vi "Lift.vi"() -> ()   [LabVIEW 2018]
uses:
  <vilib>/Rock Robotics/WPI/ThirdParty/Phoenix-LabVIEW/Motor Controller/Controls/CTRE_Phoenix_MotorControl_ControlMode.ctl
  Lift Global.vi
  Times/Times Global.vi
  <vilib>/addons/control/pid/pid.llb/PID (DBL).vi
  <vilib>/Rock Robotics/WPI/ThirdParty/Phoenix-LabVIEW/Motor Controller/Get/CTRE_Phoenix_MotorController_GetSelectedSensorData.vi
  Cargo Intake/Cargo Intake Global.vi
  <vilib>/addons/control/pid/NI_PID_pid.lvlib
  <vilib>/Rock Robotics/WPI/Counter/WPI_CounterDigitalInputToDigitalSource.vi
  <vilib>/Rock Robotics/SystemInterfaces/DIO/FPGA_DIOChannel.ctl
panel:
  in  "Zero":bool
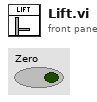
[diagram p1: front panel]
types:
  T1 = typedef "FPGA_DIOChannel.ctl" = enum8{"DIO 0", "DIO 1", "DIO 2", "DIO 3", "DIO 4", "DIO 5", "DIO 6", "DIO 7", "DIO 8", "DIO 9", "DIO MXP 0", "DIO MXP 1", "DIO MXP 2", "DIO MXP 3", "DIO MXP 4", "DIO MXP 5", "DIO MXP 6", "DIO MXP 7", "DIO MXP 8", "DIO MXP 9", "DIO MXP 10", "DIO MXP 11", "DIO MXP 12", "DIO MXP 13", "DIO MXP 14", "DIO MXP 15", "SPI Port CS1", "SPI Port CS2", "SPI Port CS3", "SPI Port MISO", "SPI Port MOSI", "Invalid"}
  T2 = typedef "WPI_DigitalInputDevRef.ctl" = cluster{"DevStatus":errorcluster, "DIO Channel":T1}
  T3 = typedef "FPGA_CounterEncoderSourceConvertionLVSourceType.ctl" = cluster{"DevStatus":errorcluster, "AnalogTriggerMode?":bool, "DigitalMode":cluster{"DIO Channel":T4}, "AnalogTriggerMode":cluster{"AnalogTriggerIndex":T5, "OutputType":T6}}
  T4 = typedef "FPGA_DIODigitalSourceChannel.ctl" = enum8{"DIO 0", "DIO 1", "DIO 2", "DIO 3", "DIO 4", "DIO 5", "DIO 6", "DIO 7", "DIO 8", "DIO 9", "DIO MXP 0", "DIO MXP 1", "DIO MXP 2", "DIO MXP 3", "DIO MXP 4", "DIO MXP 5", "DIO MXP 6", "DIO MXP 7", "DIO MXP 8", "DIO MXP 9", "DIO MXP 10", "DIO MXP 11", "DIO MXP 12", "DIO MXP 13", "DIO MXP 14", "DIO MXP 15", "SPI Port CS1", "SPI Port CS2", "SPI Port CS3", "SPI Port MISO", "SPI Port MOSI", "Disabled"}
  T5 = typedef "FPGA_AnalogTriggerIndex.ctl" = enum8{"Trig 0", "Trig 1", "Trig 2", "Trig 3", "Trig 4", "Trig 5", "Trig 6", "Trig 7", "Invalid"}
  T6 = typedef "FPGA_AnalogTriggerOutType.ctl" = enum16{"InWindow", "TriggerState", "Rising", "Falling"}
  T7 = typedef "WPI_EncoderDevRef.ctl" = cluster{"DevStatus":errorcluster, "EncoderIndex":T8, "CounterIndex":T9, "DistancePerCount":dbl, "Decoding Type":T10}
  T8 = typedef "FPGA_EncoderIdx.ctl" = enum8{"Enc 0", "Enc 1", "Enc 2", "Enc 3", "Enc 4", "Enc 5", "Enc 6", "Enc 7", "Invalid"}
  T9 = typedef "FPGA_CounterCtrSystemIndex.ctl" = enum8{"Ctr 0", "Ctr 1", "Ctr 2", "Ctr 3", "Ctr 4", "Ctr 5", "Ctr 6", "Ctr 7", "Invalid"}
  T10 = typedef "WPI_EncoderType.ctl" = enum16{"1x", "2x", "4x"}
  T11 = enum16{"Ultra Manual Control", "Manual Control", "Basic Control", "Automated Control", "Autonomous Control"}
  T12 = enum16{"N/A", "Hatch Panel Zone 1", "Hatch Panel Zone 2", "Hatch Panel Zone 3", "Cargo Zone 1", "Cargo Zone 2", "Cargo Zone 3"}
  T13 = typedef "WPI_MotorControlDeviceRef.ctl" = cluster{"DeviceStatus":errorcluster, "Type":T14, "PWM":cluster{"PWM Channel":T15, "DeadBand":T16}, "CAN":cluster{"Device Number":u8, "SetOutput VI Ref":variant, "GetOutput VI Ref":variant, "Enable VI Ref":variant, "Disable VI Ref":variant, "Data":variant}, "Invert":bool, "DIO PWM":cluster{"PWM \"Enable\" Channel":T15, "DIOChannel":T1, "PWM Rate":dbl}}
  T14 = typedef "WPI_MotorControlType.ctl" = enum16{"PWM", "CAN", "DIO PWM"}
  T15 = typedef "FPGA_DIOPWMChannel.ctl" = enum8{"PWM 0", "PWM 1", "PWM 2", "PWM 3", "PWM 4", "PWM 5", "PWM 6", "PWM 7", "PWM 8", "PWM 9", "PWM MXP 0", "PWM MXP 1", "PWM MXP 2", "PWM MXP 3", "PWM MXP 4", "PWM MXP 5", "PWM MXP 6", "PWM MXP 7", "PWM MXP 8", "PWM MXP 9", "Invalid"}
  T16 = typedef "WPI_PWMDeadband.ctl" = cluster{"Name":string, "maxPositivePwm":i32, "minPositivePwm":i32, "centerPwm":i32, "maxNegativePwm":i32, "minNegativePwm":i32, "angularRange":u16}
  T17 = typedef "CTRE_Phoenix_MotorControl_ControlMode.ctl" = u16
  T18 = typedef "Control 3.ctl" = dbl
  T19 = cluster{"proportional gain (Kc)":dbl, "integral time(Ti, min)":dbl, "derivative time(Td, min) 2":dbl}
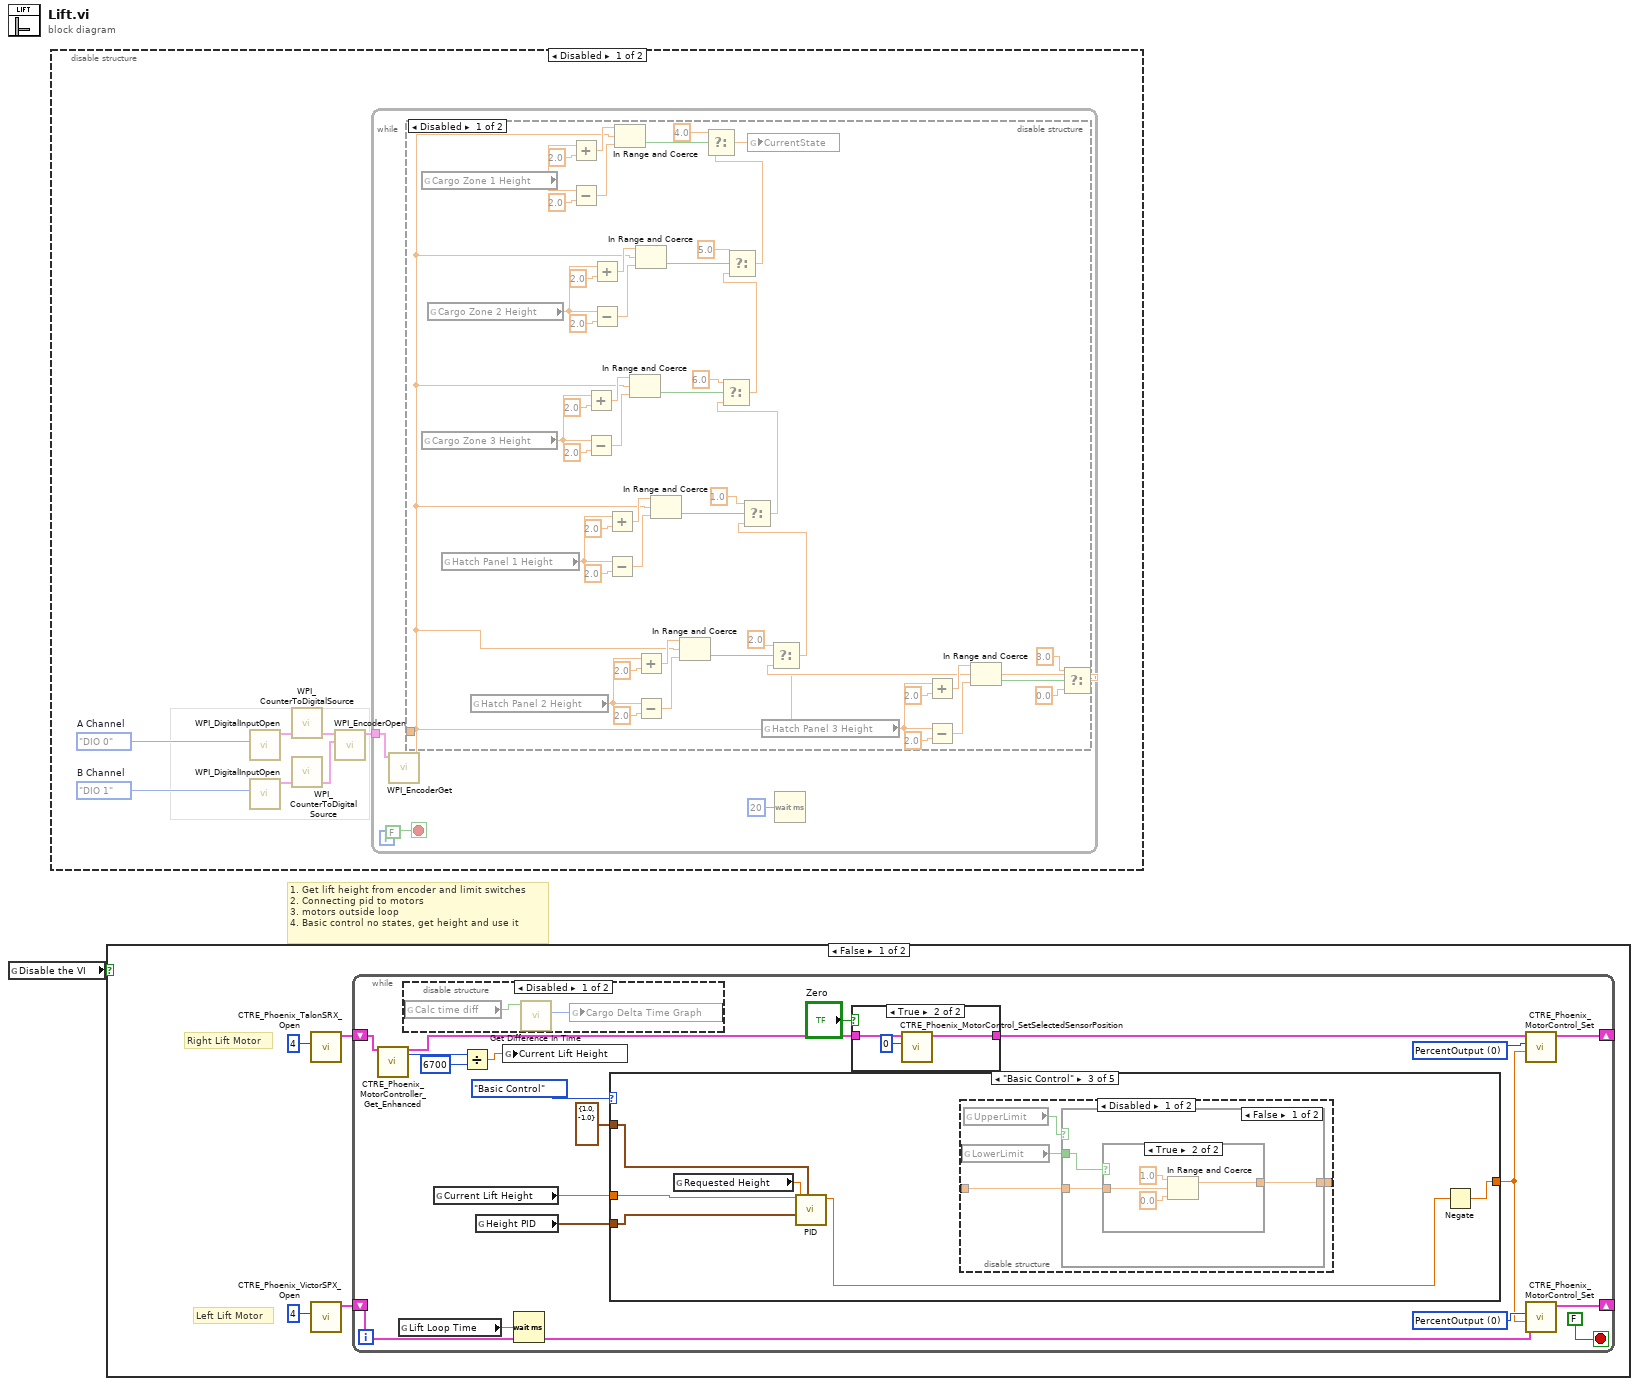
[diagram p0: block diagram]
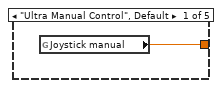
[diagram p6: hidden frame]
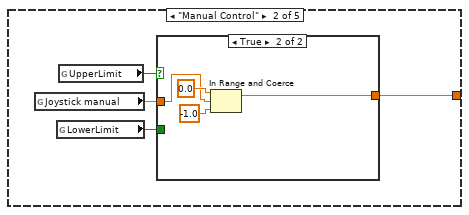
[diagram p7: hidden frame]
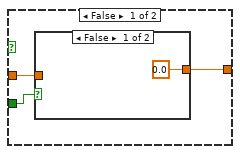
[diagram p8: hidden frame]
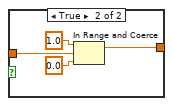
[diagram p9: hidden frame]
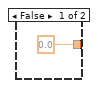
[diagram p10: hidden frame]
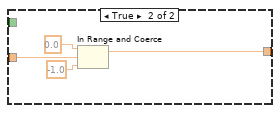
[diagram p11: hidden frame]
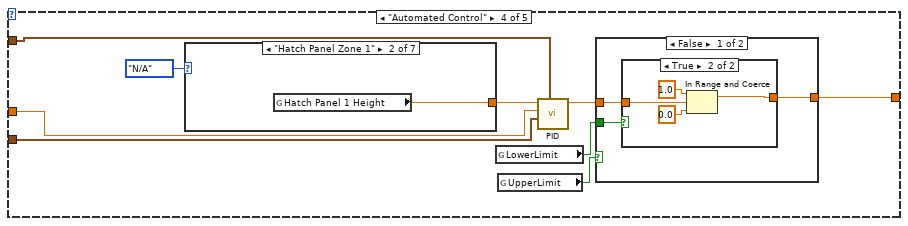
[diagram p13: hidden frame]
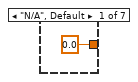
[diagram p14: hidden frame]
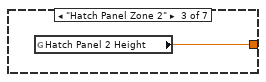
[diagram p15: hidden frame]
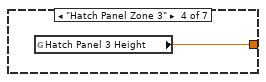
[diagram p16: hidden frame]
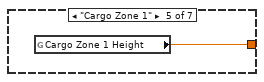
[diagram p17: hidden frame]
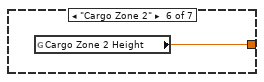
[diagram p18: hidden frame]
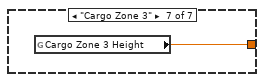
[diagram p19: hidden frame]
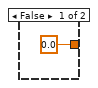
[diagram p20: hidden frame]
diagram:
  # "1. Get lift height from encoder and limit switches\n2. Connecting pid to motors\n3. motors outside loop\n4. Basic control no states, get height and use it"
  n1 = global read "Lift Global.vi" "Disable the VI"() -> (w1:bool)
  n2 = disable-structure shown="Disabled" {
    frame Disabled {
      w8 = FPGA_DIOChannel."DIO 1"  # B Channel
      w7 = FPGA_DIOChannel."DIO 0"  # A Channel
      n3 = call <vilib>:"WPI_DigitalInputOpen.vi"("DIO Channel"=w7) -> ("DigitalInputDevRef"=w4:T2)  [unwired: 1 in, 9 out]
      n4 = call <vilib>:"WPI_DigitalInputOpen.vi"("DIO Channel"=w8) -> ("DigitalInputDevRef"=w5:T2)  [unwired: 1 in, 9 out]
      n5 = call-poly <vilib>:"WPI_CounterToDigitalSource.vi"("DigitalInputDevRef"=w4) -> ("Digital Source"=w3:T3)  [unwired: 6 out]
      n6 = call-poly <vilib>:"WPI_CounterToDigitalSource.vi"("DigitalInputDevRef"=w5) -> ("Digital Source"=w6:T3)  [unwired: 6 out]
      n7 = call <vilib>:"WPI_EncoderOpen.vi"("BSource"=w6, "ASource"=w3) -> ("EncoderDevRef"=w2:T7)  [unwired: 6 in, 3 out]
      n8 = while {
        tunnel: w2 -> [w12]
        stop <- FALSE stop-if-true
        n9 = call <vilib>:"WPI_EncoderGet.vi"("EncoderDevRef"=w12) -> ("Distance"=w10:dbl)  [unwired: 5 in, 5 out]
        n10 = disable-structure shown="Disabled" {
          disable-tunnel: w10 -> [w13 _]
          frame Disabled {
            n11 = global read "Lift Global.vi" "Cargo Zone 1 Height"() -> (w53:dbl)
            n12 = global read "Lift Global.vi" "Cargo Zone 3 Height"() -> (w41:dbl)
            n13 = global read "Lift Global.vi" "Cargo Zone 2 Height"() -> (w59:dbl)
            n14 = global read "Lift Global.vi" "Hatch Panel 1 Height"() -> (w47:dbl)
            n15 = global read "Lift Global.vi" "Hatch Panel 2 Height"() -> (w29:dbl)
            n16 = Add(x=w53, y=2.0) -> (x+y=w55:dbl)
            n17 = Subtract(x=w53, y=2.0) -> (x-y=w56:dbl)
            n18 = Add(x=w41, y=2.0) -> (x+y=w43:dbl)
            n19 = Subtract(x=w41, y=2.0) -> (x-y=w44:dbl)
            n20 = Add(x=w59, y=2.0) -> (x+y=w61:dbl)
            n21 = Subtract(x=w59, y=2.0) -> (x-y=w62:dbl)
            n22 = Add(x=w47, y=2.0) -> (x+y=w49:dbl)
            n23 = Subtract(x=w47, y=2.0) -> (x-y=w50:dbl)
            n24 = In Range and Coerce(upper limit=w55, x=w13, lower limit=w56) -> (In Range?=w51:bool)  [unwired: 1 out]
            n25 = In Range and Coerce(upper limit=w43, x=w13, lower limit=w44) -> (In Range?=w39:bool)  [unwired: 1 out]
            n26 = In Range and Coerce(upper limit=w61, x=w13, lower limit=w62) -> (In Range?=w57:bool)  [unwired: 1 out]
            n27 = Add(x=w29, y=2.0) -> (x+y=w31:dbl)
            n28 = Subtract(x=w29, y=2.0) -> (x-y=w32:dbl)
            n29 = In Range and Coerce(upper limit=w49, x=w13, lower limit=w50) -> (In Range?=w45:bool)  [unwired: 1 out]
            n30 = In Range and Coerce(upper limit=w31, x=w13, lower limit=w32) -> (In Range?=w27:bool)  [unwired: 1 out]
            n31 = global read "Lift Global.vi" "Hatch Panel 3 Height"() -> (w35:dbl)
            n32 = Add(x=w35, y=2.0) -> (x+y=w37:dbl)
            n33 = Subtract(x=w35, y=2.0) -> (x-y=w38:dbl)
            n34 = In Range and Coerce(upper limit=w37, x=w13, lower limit=w38) -> (In Range?=w33:bool)  [unwired: 1 out]
            n35 = Select(t=3.0, s=w33, f=0.0 ("t")) -> (s? t:f=w23:dbl)
            n36 = Select(t=2.0, s=w27, f=w23) -> (s? t:f=w24:dbl)
            n37 = Select(t=1.0, s=w45, f=w24) -> (s? t:f=w25:dbl)
            n38 = Select(t=6.0, s=w39, f=w25) -> (s? t:f=w26:dbl)
            n39 = Select(t=5.0, s=w57, f=w26) -> (s? t:f=w20:dbl)
            n40 = Select(t=4.0, s=w51, f=w20) -> (s? t:f=w21:dbl)
            n41 = global write "Lift Global.vi" "CurrentState"(w21) -> ()
          }
          frame Enabled {
          }
        }
        n42 = Wait (ms)(milliseconds to wait=u32 20) -> ()  [unwired: 1 out]
      }
    }
    frame Enabled {
    }
  }
  n43 = case shown="False" w1 {
    frame False {
      # "Left Lift Motor"
      # "Right Lift Motor"
      n44 = call <vilib>:"CTRE_Phoenix_TalonSRX_Open.vi"("Device Number"=u8 4) -> ("CAN Talon SRX Ref"=w66:T13)  [unwired: 9 in, 1 out]
      n45 = call <vilib>:"CTRE_Phoenix_VictorSPX_Open.vi"("Device Number"=u8 4) -> ("CAN Talon SRX Ref"=w64:T13)  [unwired: 9 in, 1 out]
      n46 = while {
        shift-right: [w81] -> _
        shift-left: w66 -> [w73]
        shift-right: [w79] -> _
        shift-left: w64 -> [w78]
        stop <- FALSE stop-if-true
        w80 = T17 0 items=["PercentOutput"=0, "Position"=1, "Velocity"=2, "Current"=3, "Follower"=5, "MotionProfile"=6, "MotionMagic"=7, "MotionProfileArc"=10, "Disabled"=15] ("Control Mode")
        w82 = T17 0 items=["PercentOutput"=0, "Position"=1, "Velocity"=2, "Current"=3, "Follower"=5, "MotionProfile"=6, "MotionMagic"=7, "MotionProfileArc"=10, "Disabled"=15] ("Control Mode")
        n47 = call-poly <vilib>:"CTRE_Phoenix_MotorController_Get_Enhanced.vi"("PhoenixMotorControlDevRef"=w73) -> ("PhoenixMotorControlDevRef"=w72:T13, "Position (Raw Sensor Units)"=w69:i32)  [unwired: 11 in, 2 out]
        n48 = global read "Times Global.vi" "Lift Loop Time"() -> (w85:T18)
        n49 = disable-structure shown="Disabled" {
          frame Disabled {
            n50 = global read "Cargo Intake Global.vi" "Calc time diff"() -> (w91:bool)
            n51 = call "Get Difference In Time.vi"("Calculate Time Difference"=w91) -> ("Delta Time over Time"=w90:u32)  [unwired: 9 in, 1 out]
            n52 = global write "Times Global.vi" "Cargo Delta Time Graph"(w90) -> ()
          }
          frame Enabled {
          }
        }
        n53 = global read "Lift Global.vi" "Current Lift Height"() -> (w74:dbl)
        n54 = Divide(x=w69, y=6700) -> (x/y=w68:dbl)
        n55 = global read "Lift Global.vi" "Height PID"() -> (w75:T19)
        n56 = global write "Lift Global.vi" "Current Lift Height"(w68) -> ()
        n57 = Wait (ms)(milliseconds to wait=w85) -> ()  [unwired: 1 out]
        n58 = case shown="\"Basic Control\"" T11."Basic Control" ("LiftMode") {
          tunnel: [w92 w93 w110 w136 0.0 ("Cargo Zone 3 Height")] -> w77
          tunnel: w74 -> [_ _ w114 w134 _]
          tunnel: w75 -> [_ _ w113 w133 _]
          tunnel: cluster{"output high":dbl, "output low":dbl} {"output high"=1.0, "output low"=-1.0} ("output range") -> [_ _ w112 w135 _]
          frame "Ultra Manual Control", Default {
            n59 = global read "Lift Global.vi" "Joystick manual"() -> (w92:dbl)
          }
          frame "Manual Control" {
            n60 = global read "Lift Global.vi" "Joystick manual"() -> (w94:dbl)
            n61 = global read "Lift Global.vi" "LowerLimit"() -> (w96:bool)
            n62 = global read "Lift Global.vi" "UpperLimit"() -> (w95:bool)
            n63 = case shown="True" w95 {
              tunnel: w96 -> [w99 _]
              tunnel: [w98 w106] -> w93
              tunnel: w94 -> [w97 w105]
              frame False {
                n64 = case shown="False" w99 {
                  tunnel: [0.0 w104] -> w98
                  tunnel: w97 -> [_ w101]
                  frame False {
                  }
                  frame True {
                    n65 = In Range and Coerce(upper limit=1.0, x=w101, lower limit=0.0) -> (coerced(x)=w104:dbl)  [unwired: 1 out]
                  }
                }
              }
              frame True {
                n66 = In Range and Coerce(upper limit=0.0, x=w105, lower limit=-1.0) -> (coerced(x)=w106:dbl)  [unwired: 1 out]
              }
            }
          }
          frame "Basic Control" {
            n67 = global read "Lift Global.vi" "Requested Height"() -> (w111:dbl)
            n68 = call-poly <vilib>:"PID.vi"("output range"=w112, "PID gains"=w113, "process variable"=w114, "setpoint"=w111) -> ("output"=w109:dbl)  [unwired: 6 in, 1 out]
            n69 = disable-structure shown="Disabled" {
              disable-tunnel: _ -> [w116 _]
              disable-tunnel: [w115 _] -> _
              frame Disabled {
                n70 = global read "Lift Global.vi" "LowerLimit"() -> (w118:bool)
                n71 = global read "Lift Global.vi" "UpperLimit"() -> (w117:bool)
                n72 = case shown="False" w117 {
                  tunnel: w118 -> [w121 _]
                  tunnel: [w120 w128] -> w115
                  tunnel: w116 -> [w119 w127]
                  frame False {
                    n73 = case shown="True" w121 {
                      tunnel: [0.0 w126] -> w120
                      tunnel: w119 -> [_ w123]
                      frame False {
                      }
                      frame True {
                        n74 = In Range and Coerce(upper limit=1.0, x=w123, lower limit=0.0) -> (coerced(x)=w126:dbl)  [unwired: 1 out]
                      }
                    }
                  }
                  frame True {
                    n75 = In Range and Coerce(upper limit=0.0, x=w127, lower limit=-1.0) -> (coerced(x)=w128:dbl)  [unwired: 1 out]
                  }
                }
              }
              frame Enabled {
              }
            }
            n76 = Negate(x=w109) -> (-x=w110:dbl)
          }
          frame "Automated Control" {
            n77 = case shown="\"Hatch Panel Zone 1\"" T12."N/A" ("LiftLocation") {
              tunnel: [0.0 ("Cargo Zone 3 Height") w141 w142 w143 w144 w145 w146] -> w131
              frame "N/A", Default {
              }
              frame "Hatch Panel Zone 1" {
                n78 = global read "Lift Global.vi" "Hatch Panel 1 Height"() -> (w141:dbl)
              }
              frame "Hatch Panel Zone 2" {
                n79 = global read "Lift Global.vi" "Hatch Panel 2 Height"() -> (w142:dbl)
              }
              frame "Hatch Panel Zone 3" {
                n80 = global read "Lift Global.vi" "Hatch Panel 3 Height"() -> (w143:dbl)
              }
              frame "Cargo Zone 1" {
                n81 = global read "Lift Global.vi" "Cargo Zone 1 Height"() -> (w144:dbl)
              }
              frame "Cargo Zone 2" {
                n82 = global read "Lift Global.vi" "Cargo Zone 2 Height"() -> (w145:dbl)
              }
              frame "Cargo Zone 3" {
                n83 = global read "Lift Global.vi" "Cargo Zone 3 Height"() -> (w146:dbl)
              }
            }
            n84 = global read "Lift Global.vi" "LowerLimit"() -> (w139:bool)
            n85 = global read "Lift Global.vi" "UpperLimit"() -> (w138:bool)
            n86 = call-poly <vilib>:"PID.vi"("output range"=w135, "PID gains"=w133, "process variable"=w134, "setpoint"=w131) -> ("output"=w137:dbl)  [unwired: 6 in, 1 out]
            n87 = case shown="False" w138 {
              tunnel: w139 -> [w149 _]
              tunnel: [w148 w156] -> w136
              tunnel: w137 -> [w147 w155]
              frame False {
                n88 = case shown="True" w149 {
                  tunnel: [0.0 w154] -> w148
                  tunnel: w147 -> [_ w151]
                  frame False {
                  }
                  frame True {
                    n89 = In Range and Coerce(upper limit=1.0, x=w151, lower limit=0.0) -> (coerced(x)=w154:dbl)  [unwired: 1 out]
                  }
                }
              }
              frame True {
                n90 = In Range and Coerce(upper limit=0.0, x=w155, lower limit=-1.0) -> (coerced(x)=w156:dbl)  [unwired: 1 out]
              }
            }
          }
          frame "Autonomous Control" {
          }
        }
        n91 = case shown="True" "Zero" {
          tunnel: w72 -> [w86 w89]
          tunnel: [w86 w88] -> w71
          frame False {
          }
          frame True {
            n92 = call <vilib>:"CTRE_Phoenix_MotorControl_SetSelectedSensorPosition.vi"("New Sensor Position"=0, "PhoenixMotorControlDevRef"=w89) -> ("PhoenixMotorControlDevRef"=w88:T13)  [unwired: 8 in, 1 out]
          }
        }
        n93 = call <vilib>:"CTRE_Phoenix_MotorControl_Set.vi"("Output"=w77, "Control Mode"=w82, "PhoenixMotorControlDevRef"=w71) -> ("PhoenixMotorControlDevRef"=w81:T13)  [unwired: 7 in, 1 out]
        n94 = call <vilib>:"CTRE_Phoenix_MotorControl_Set.vi"("Output"=w77, "Control Mode"=w80, "PhoenixMotorControlDevRef"=w78) -> ("PhoenixMotorControlDevRef"=w79:T13)  [unwired: 7 in, 1 out]
      }
    }
    frame True {
    }
  }
